vi "SDCCB Test Panel.vi"() -> ()   [LabVIEW 2020]
uses:
  <vilib>/Utility/error.llb/whitespace.ctl
  <vilib>/Instr/_visa.llb/VISA Configure Serial Port (Instr).vi
panel:
  out "Firmware Version":string
  in  "COM Port":refnum<visa-resource-name>
  out "Connected":bool
  out "Waiting for Reply":bool
  out "Last Error":errorcluster
  out "Command History":string
  out "Reply":string
  in  "Command":string
  in  "Quit":bool
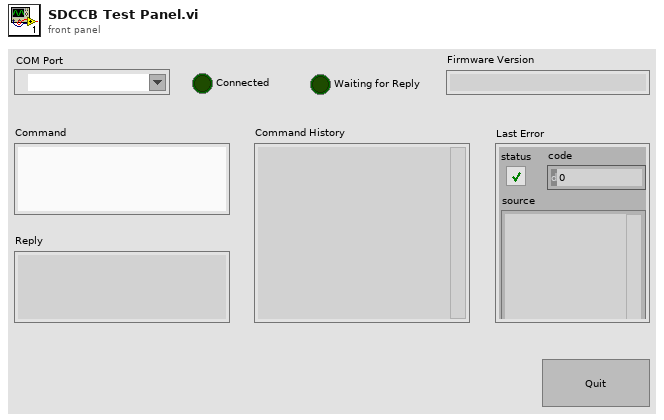
[diagram p1: front panel]
types:
  T1 = typedef "whitespace.ctl" = u16
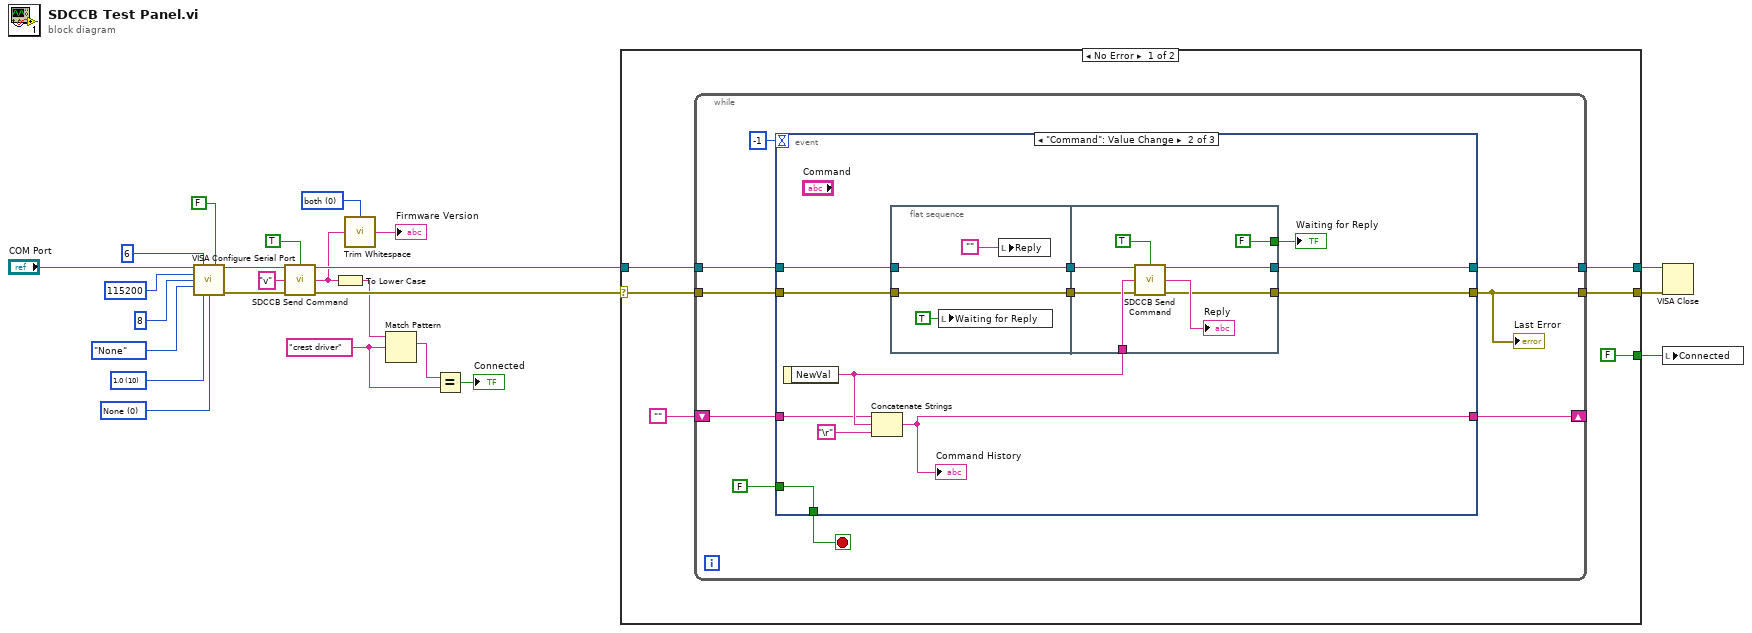
[diagram p0: block diagram]
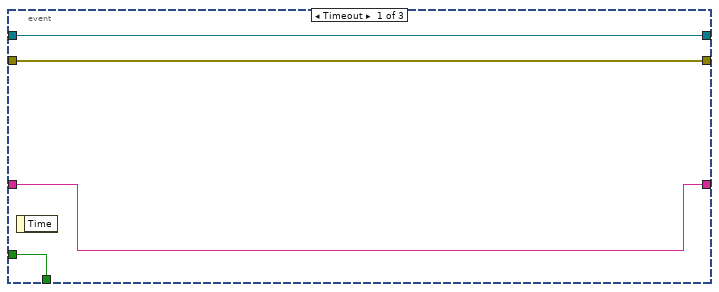
[diagram p2: hidden frame]
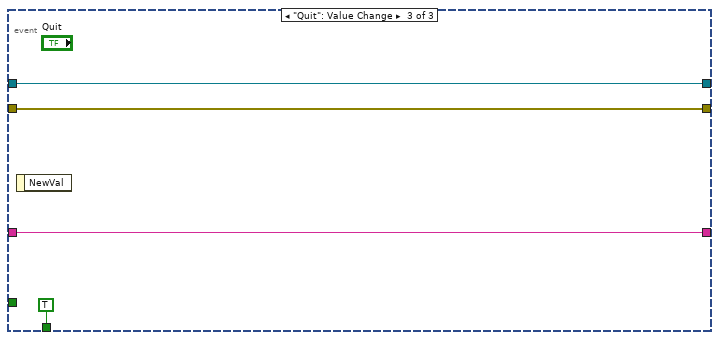
[diagram p3: hidden frame]
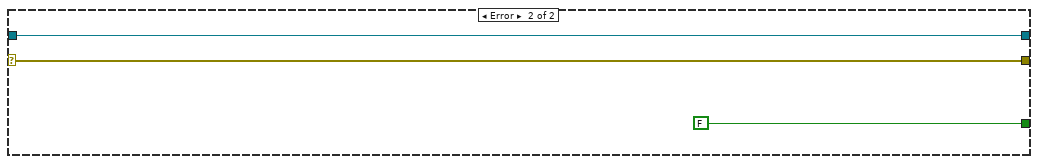
[diagram p4: hidden frame]
diagram:
  w1 = T1 0 items=["both", "start of string", "end of string"] ("location (both)")
  w5 = "crest driver"
  w16 = u16 0 items=["None", "XON/XOFF", "RTS/CTS", "XON/XOFF & RTS/CTS", "DTR/DSR", "XON/XOFF & DTR/DSR"] ("flow control (0:none)")
  w17 = u16 10 items=["1.0"=10, "1.5"=15, "2.0"=20] ("stop bits (10: 1 bit)")
  n1 = call-poly "VISA Configure Serial Port"("VISA resource name"="COM Port", "timeout (10sec)"=u32 6, "Enable Termination\nChar (T)"=FALSE ("Enable Termination\nChar (T)"), "baud rate (9600)"=u32 115200, "data bits (8)"=u16 8, "parity (0:none)"=enum16{"None", "Odd", "Even", "Mark", "Space"}."None", "stop bits (10: 1 bit)"=w17, "flow control (0:none)"=w16) -> ("VISA resource name out"=w13:refnum<visa-resource-name>, "error out"=w12:errorcluster)  [unwired: 6 in]
  n2 = call "SDCCB Send Command.vi"("VISA Ref"=w13, "Wait for Reply (T)"=TRUE, "Command"="v", "Error In"=w12) -> ("VISA Ref Dup"=w10:refnum<visa-resource-name>, "Reply"=w3:string, "Error Out"=w9:errorcluster)  [unwired: 9 in]
  n3 = To Lower Case(string=w3) -> (all lower case string=w7:string)
  n4 = call <vilib>:"Trim Whitespace.vi"("string"=w3, "location (both)"=w1) -> ("trimmed string"=→"Firmware Version":string)
  n5 = Match Pattern(string=w7, regular expression=w5) -> (match substring=w6:string)  [unwired: 1 in, 3 out]
  n6 = Equal?(x=w6, y=w5) -> (x = y?=→"Connected":bool)
  n7 = case shown="No Error" w9 {
    selector: w9 -> [w29 w73]
    tunnel: w10 -> [w30 w74]
    tunnel: [w28 w74] -> w24
    tunnel: [w27 w73] -> w23
    tunnel: [FALSE FALSE] -> w22
    frame No Error {
      n8 = while {
        tunnel: w30 -> [w37]
        tunnel: w29 -> [w36]
        tunnel: [w35] -> w28
        tunnel: [w32] -> w27
        shift-right: [w33] -> _
        shift-left: "" -> [w34]
        stop <- w38 stop-if-true
        n9 = event shown="[1] \"Command\": Value Change" {
          selector: _ -> [_ _ _]
          dyn-events: _ -> [_ _ _]
          timeout: -1 -> [_ _ _]
          tunnel: FALSE -> [w43 w55 _]
          tunnel: [w43 w55 TRUE] -> w38
          tunnel: w37 -> [w41 w54 w71]
          tunnel: w36 -> [w40 w53 w70]
          tunnel: [w41 w49 w71] -> w35
          tunnel: [w40 w50 w70] -> w32
          tunnel: w34 -> [w42 w46 w68]
          tunnel: [w42 w45 w68] -> w33
          event Timeout {
            n10 = event-data() -> ()  [unwired: 1 in, 1 out]
          }
          event "Command": Value Change {
            n11 = event-data() -> ("NewVal"=w48:string)  [unwired: 1 in]
            n12 = Concatenate Strings(w46, w48, "\r") -> (w45:string)
            "Command History" <- w45
            n13 = flat-sequence {
              tunnel: w53 -> [w58]
              tunnel: w54 -> [w59]
              tunnel: [w59] -> w52
              tunnel: [w58] -> w51
              tunnel: w48 -> [w66]
              tunnel: w52 -> [w67]
              tunnel: w51 -> [w65]
              tunnel: [w63] -> w50
              tunnel: [w62] -> w49
              tunnel: [FALSE] -> w44
              frame #0 {
                n14 = local write "Waiting for Reply"(TRUE ("Waiting for Cmd")) -> ()
                n15 = local write "Reply"("") -> ()
              }
              frame #1 {
                n16 = call "SDCCB Send Command.vi"("VISA Ref"=w67, "Wait for Reply (T)"=TRUE, "Command"=w66, "Error In"=w65) -> ("VISA Ref Dup"=w62:refnum<visa-resource-name>, "Reply"=→"Reply":string, "Error Out"=w63:errorcluster)  [unwired: 9 in]
              }
            }
            "Waiting for Reply" <- w44
          }
          event "Quit": Value Change {
            n17 = event-data() -> ()  [unwired: 1 in, 1 out]
          }
        }
        "Last Error" <- w32
      }
    }
    frame Error {
    }
  }
  n18 = VISA Close(VISA resource name=w24, error in (no error)=w23) -> ()  [unwired: 1 out]
  n19 = local write "Connected"(w22) -> ()
